vi "createSketch.vi"(11 "path to ino folder":path) -> (3 "path to sketch folder":path)   [LabVIEW 2020]
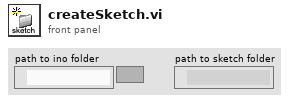
[diagram p1: front panel]
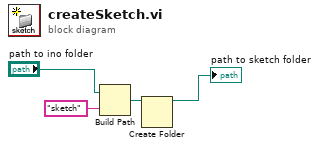
[diagram p0: block diagram]
diagram:
  n1 = Build Path(base path="path to ino folder", name or relative path="sketch") -> (appended path=w2:path)
  n2 = Create Folder(path (use dialog)=w2) -> (created path=→"path to sketch folder":path)  [unwired: 2 in, 2 out]
